vi "shared-dependency-staticallydefined-test.vi"(8 "error in (no error)":errorcluster) -> (0 "error out":errorcluster)   [LabVIEW 2013]
uses:
  _test-support-SMOs/SMO.C/SMO.C.lvclass
  _test-support-SMOs/SMO.D/SMO.D.lvclass
  src/SMO/SMO.lvclass
  <vilib>/addons/_JKI Toolkits/Caraya/classes/Assert/Assert.lvclass
  <vilib>/addons/_JKI Toolkits/Caraya/classes/Test/Test.lvclass
panel:
  out "size(s) 2":i32
  out "size(s)":i32
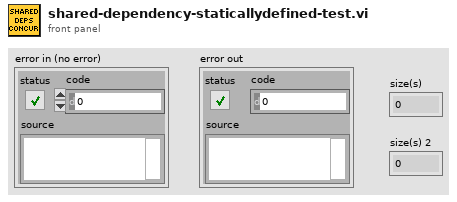
[diagram p1: front panel]
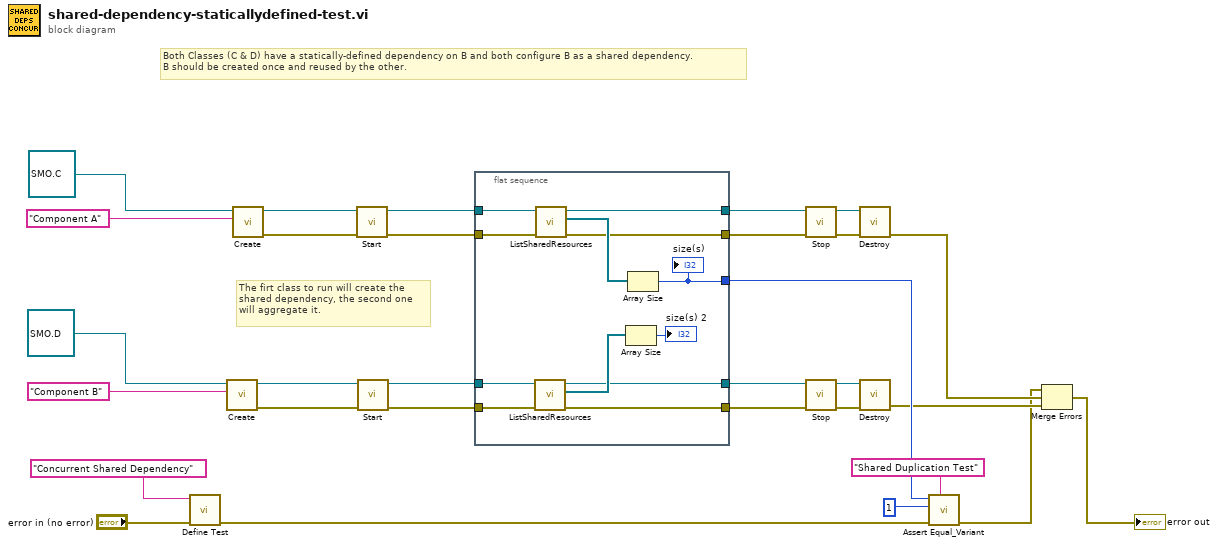
[diagram p0: block diagram]
diagram:
  # "Both Classes (C & D) have a statically-defined dependency on B and both configure B as a shared dependency.\nB should be created once and reused by the other."
  # "The firt class to run will create the\nshared dependency, the second one\nwill aggregate it."
  n1 = call <vilib>:"Define Test.vi"("error in (no error)"="error in (no error)", "Label (VI Title)"="Concurrent Shared Dependency") -> ("error out"=w7:errorcluster)  [unwired: 9 in]
  n2 = call "Create.vi"("Subsystem Name (optional)"="Component B", "SMO"=refnum<class "SMO.D.lvclass"> refnum ("SMO.D.lvclass")) -> ("error out"=w3:errorcluster, "SMO out"=w19:refnum<class "SMO.D.lvclass">)  [unwired: 7 in, 1 out]
  n3 = call "Create.vi"("Subsystem Name (optional)"="Component A", "SMO"=refnum<class "SMO.C.lvclass"> refnum ("SMO.C.lvclass")) -> ("error out"=w4:errorcluster, "SMO out"=w15:refnum<class "SMO.C.lvclass">)  [unwired: 7 in, 1 out]
  n4 = call "Start.vi"("error in (no error)"=w4, "SMO"=w15) -> ("error out"=w2:errorcluster, "SMO out"=w24:refnum<class "SMO.C.lvclass">)  [unwired: 8 in]
  n5 = call "Start.vi"("error in (no error)"=w3, "SMO"=w19) -> ("error out"=w1:errorcluster, "SMO out"=w25:refnum<class "SMO.D.lvclass">)  [unwired: 8 in]
  n6 = flat-sequence {
    tunnel: [w42] -> w29
    tunnel: [w40] -> w28
    tunnel: [w32] -> w27
    tunnel: [w34] -> w26
    tunnel: w1 -> [w33]
    tunnel: w25 -> [w35]
    tunnel: w2 -> [w39]
    tunnel: w24 -> [w38]
    tunnel: [w37] -> w6
    frame #0 {
      n7 = call "ListSharedResources.vi"("error in (no error)"=w33, "SMO in"=w35) -> ("error out"=w32:errorcluster, "Shared Resources"=w36:refnum<class "SMO.lvclass">[], "SMO out"=w34:refnum<class "SMO.D.lvclass">)  [unwired: 6 in, 1 out]
      n8 = call "ListSharedResources.vi"("error in (no error)"=w39, "SMO in"=w38) -> ("error out"=w37:errorcluster, "Shared Resources"=w41:refnum<class "SMO.lvclass">[], "SMO out"=w40:refnum<class "SMO.C.lvclass">)  [unwired: 6 in, 1 out]
      n9 = Array Size(array=w36) -> (size(s)=→"size(s) 2":i32)
      n10 = Array Size(array=w41) -> (size(s)=w42:i32)
      "size(s)" <- w42
    }
  }
  n11 = call "Stop.vi"("error in (no error)"=w6, "SMO"=w28) -> ("error out"=w18:errorcluster, "SMO out"=w17:refnum<class "SMO.C.lvclass">)  [unwired: 8 in]
  n12 = call "Stop.vi"("error in (no error)"=w27, "SMO"=w26) -> ("error out"=w20:errorcluster, "SMO out"=w21:refnum<class "SMO.D.lvclass">)  [unwired: 8 in]
  n13 = call "Destroy.vi"("error in (no error)"=w18, "SMO"=w17) -> ("error out"=w23:errorcluster)  [unwired: 9 in]
  n14 = call "Destroy.vi"("error in (no error)"=w20, "SMO"=w21) -> ("error out"=w22:errorcluster)  [unwired: 9 in]
  n15 = call <vilib>:"Assert Equal_Variant.vi"("Label"="Shared Duplication Test" ("Filter (regex|name)"), "error in (no error)"=w7, "Y"=1, "X"=w29) -> ("error out"=w13:errorcluster)  [unwired: 7 in]
  n16 = Merge Errors(w13, w23, w22) -> (→"error out":errorcluster)
